vi "Destroy_MsgQ.vi"(8 "error in (no error)":errorcluster) -> (0 "error out":errorcluster)   [LabVIEW 2019, in "MsgQ.lvlib"]
uses:
  MsgQ.lvlib
  TypeDefs/CommandsQ.ctl
  TypeDefs/MsgQ_Commands.ctl
  mmw_Service/Service.lvlib
  mmw_Service/TypeDef/NotifierQ.ctl
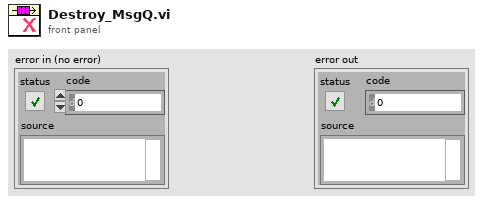
[diagram p1: front panel]
types:
  T1 = typedef "Service.lvlib/CommandsQ.ctl" = cluster{"cmd":T2, "data":variant, "notif":string}
  T2 = typedef "MsgQ.lvlib/MsgQ_Commands.ctl" = enum16{"message1", "message2", "message3", "generic", "transparent", "exception", "stop"}
  T3 = typedef "Service.lvlib/NotifierQ.ctl" = cluster{"Data":variant, "Code":dbl}
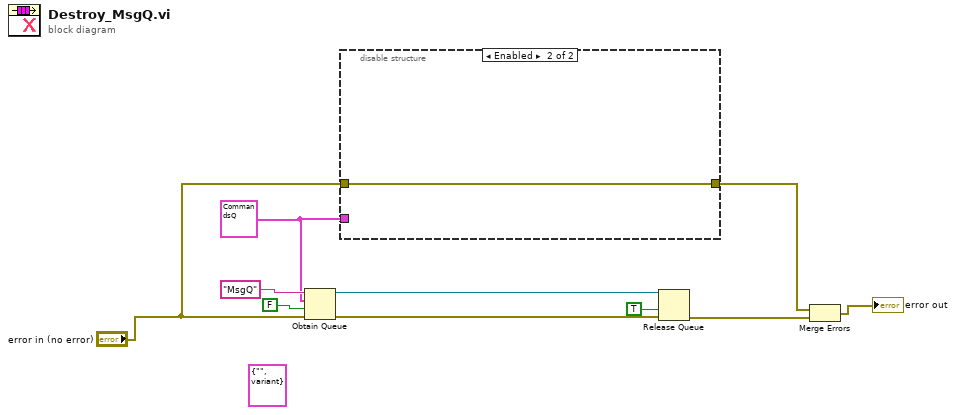
[diagram p0: block diagram]
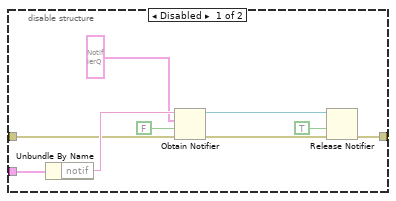
[diagram p2: hidden frame]
diagram:
  w5 = T1 {"cmd"=enum."message1", "data"=variant, "notif"="notif1"}
  (unwired) cluster{enum16{""}, "element data type":variant} {enum."", "element data type"=variant}
  n1 = Obtain Queue(name (unnamed)="MsgQ", element data type=w5, create if not found? (T)=FALSE, error in (no error)="error in (no error)") -> (queue out=w7:refnum<queue>, error out=w6:errorcluster)  [unwired: 1 in, 1 out]
  n2 = disable-structure shown="Enabled" {
    disable-tunnel: w5 -> [w19 _]
    disable-tunnel: "error in (no error)" -> [w15 w20]
    disable-tunnel: [w11 w20] -> w3
    frame Disabled {
      n3 = Unbundle By Name(w19) -> ("notif"=w18:string)
      n4 = Obtain Notifier(name (unnamed)=w18, notification data type=T3 {"Data"=variant(enum16{""} enum.""), "Code"=0.0}, create if not found? (T)=FALSE, error in (no error)=w15) -> (notifier out=w12:refnum<notifier>, error out=w14:errorcluster)  [unwired: 1 out]
      n5 = Release Notifier(notifier=w12, force destroy? (F)=TRUE, error in (no error)=w14) -> (error out=w11:errorcluster)  [unwired: 2 out]
    }
    frame Enabled {
    }
  }
  n6 = Release Queue(queue=w7, force destroy? (F)=TRUE, error in (no error)=w6) -> (error out=w2:errorcluster)  [unwired: 2 out]
  n7 = Merge Errors(w3, w2) -> (→"error out":errorcluster)
